vi "IMAQdx Stop Acquisition.vi"(8 "error in":errorcluster, 11 "Session In":T1) -> (0 "error out":errorcluster, 3 "Session Out":T1)   [LabVIEW 2013, in "NI_Vision_Acquisition_Software.lvlib"]
doc: "Stops an acquisition previously started with IMAQdx Start Acquisition.vi."
uses:
  NI_Vision_Acquisition_Software.lvlib
  IMAQdx.ctl
  niimaqdx.dll
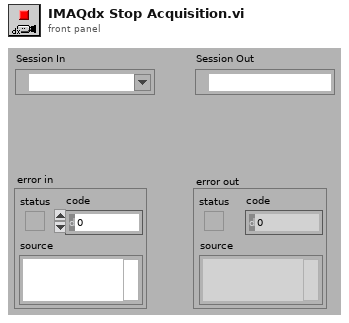
[diagram p1: front panel]
types:
  T1 = typedef "IMAQdx.ctl" = refnum<k21>
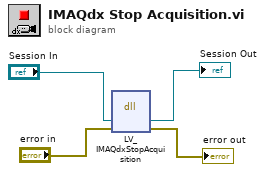
[diagram p0: block diagram]
diagram:
  n1 = dll-call lib="niimaqdx.dll" fn="LV_IMAQdxStopAcquisition"("Session In"="Session In", "error in"="error in") -> ("Session In"=→"Session Out":T1, "error in"=→"error out":errorcluster)  [unwired: 4 in, 2 out]
